vi "initialize Session Data.vi"(0 "Session in":refnum<class "Template Session.lvclass">, 11 "error in":errorcluster) -> (4 "Session out":refnum<class "Template Session.lvclass">, 15 "error out":errorcluster)   [LabVIEW 2020, in "Template Session.lvclass"]
uses:
  <userlib>/_Session Fwk/Template Session/Template Session.lvclass
  <userlib>/_Session Fwk/Session - Root.lvclass
  C:/Program Files (x86)/National Instruments/LabVIEW 2020/user.lib/_Session Fwk/Session - Root.lvclass
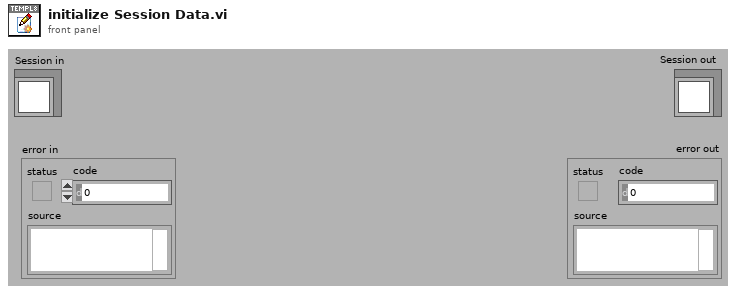
[diagram p1: front panel]
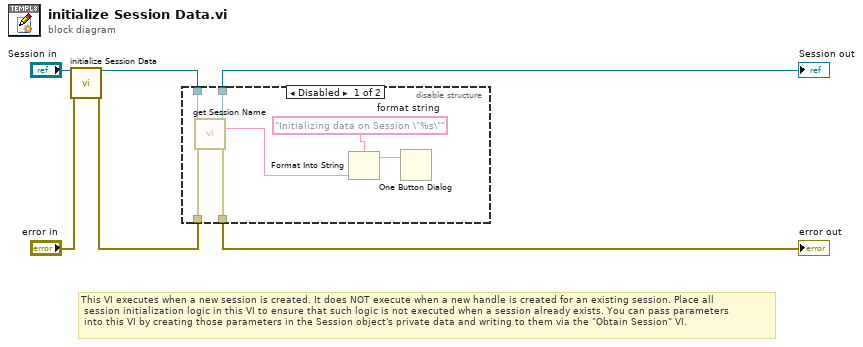
[diagram p0: block diagram]
diagram:
  # "This VI executes when a new session is created. It does NOT execute when a new handle is created for an existing session. Place all\n session initialization logic in this VI to ensure that such logic is not executed when a session already exists. You can pass parameters\n into this VI by creating those parameters in the Session object's private data and writing to them via the \"Obtain Session\" VI."
  n1 = call-parent "initialize Session Data.vi"("OBJ - Session in"="Session in", "error in"="error in") -> ("OBJ - Session out"=w3:refnum<class "Template Session.lvclass">, "error out"=w1:errorcluster)  [unwired: 12 in]
  n2 = disable-structure shown="Disabled" {
    disable-tunnel: w3 -> [w13 w15]
    disable-tunnel: [w12 w15] -> w5
    disable-tunnel: w1 -> [w8 w14]
    disable-tunnel: [w7 w14] -> w6
    frame Disabled {
      w10 = "Initializing data on Session \"%s\""  # format string
      n3 = call <userlib>:"get Session Name.vi"("OBJ - Session in"=w13, "error in (no error)"=w8) -> ("OBJ - Session out"=w12:refnum<class "Template Session.lvclass">, "Session Name"=w11:string, "error out"=w7:errorcluster)  [unwired: 11 in]
      n4 = Format Into String(format string=w10, w11) -> (resulting string=w9:string)  [unwired: 2 in, 1 out]
      n5 = One Button Dialog(message=w9) -> ()  [unwired: 1 in, 1 out]
    }
    frame Enabled {
    }
  }
  "error out" <- w6
  "Session out" <- w5
